vi "Define Default Prefix.vi"(8 "error in (no error)":errorcluster, 11 "DO Channel in":refnum<class "DO Channel.lvclass">) -> (0 "error out":errorcluster, 3 "DO Channel out":refnum<class "DO Channel.lvclass">)   [LabVIEW 2020, in "Scan Engine Scripting.lvlib" / "DO Channel.lvclass"]
uses:
  DO Channel.lvclass
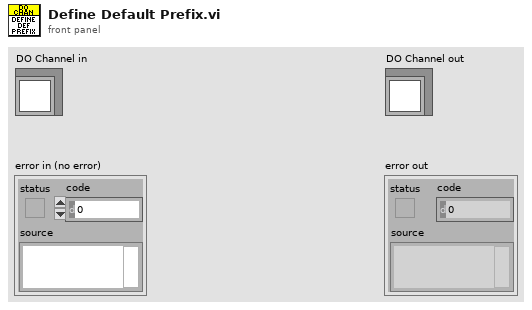
[diagram p1: front panel]
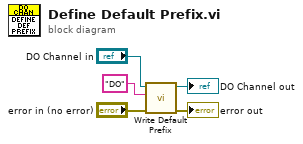
[diagram p0: block diagram]
diagram:
  n1 = call-dynamic "Write Default Prefix.vi"("error in"="error in (no error)", "default prefix"="DO", "channel in"="DO Channel in") -> ("error out"=→"error out":errorcluster, "channel out"=→"DO Channel out":refnum<class "DO Channel.lvclass">)  [unwired: 7 in]
